vi "Virt.OSC.SUBVI.vi"(0 "VISA resource name":refnum<visa-resource-name>, 11 "Error In":errorcluster) -> (2 "Channel 1 Scale":dbl, 3 "Channel 2 Scale":dbl, 4 "VISA resource name out":refnum<visa-resource-name>, 6 "Time Base":dbl, 8 "vertical trigger":dbl, 10 "horziontal trigger":dbl, 14 "rise/fall":string, 15 "Error Out":errorcluster)   [LabVIEW 2017]
uses:
  <instrlib>/Tektronix TDS 200 1000 2000 Series/Tektronix TDS 200 1000 2000 Series.lvlib
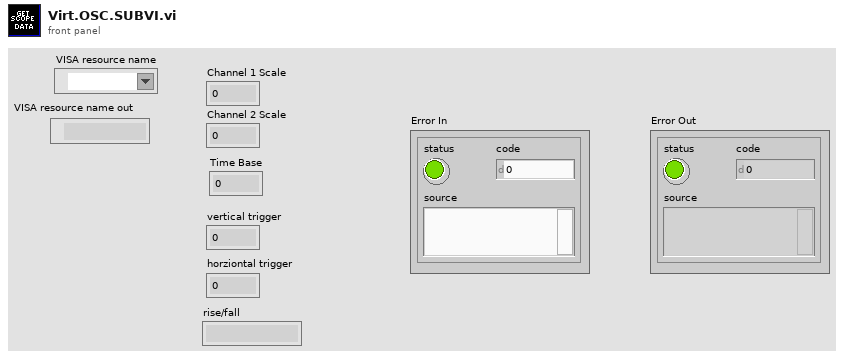
[diagram p1: front panel]
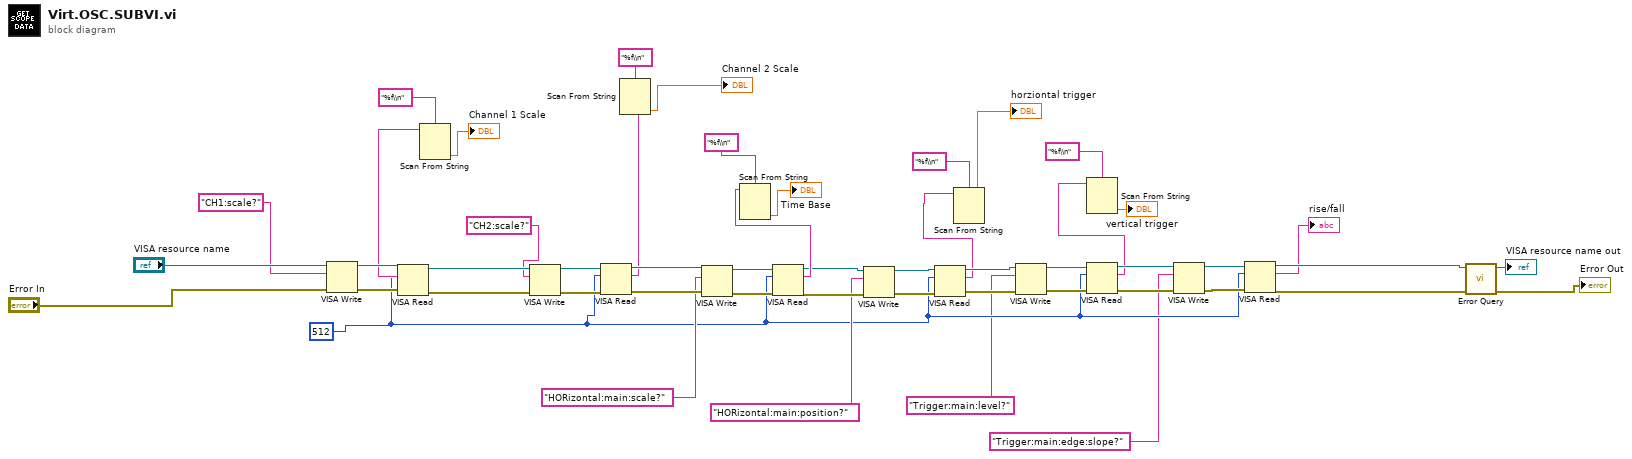
[diagram p0: block diagram]
diagram:
  w10 = 512
  n1 = VISA Write(VISA resource name="VISA resource name", write buffer="CH1:scale?" ("format string"), error in (no error)="Error In") -> (VISA resource name out=w44:refnum<visa-resource-name>, error out=w39:errorcluster)  [unwired: 1 out]
  n2 = VISA Read(VISA resource name=w44, byte count=w10, error in (no error)=w39) -> (VISA resource name out=w43:refnum<visa-resource-name>, read buffer=w34:string, error out=w38:errorcluster)  [unwired: 1 out]
  n3 = Scan From String(format string="%f\\n", input string=w34) -> (output 1=→"Channel 1 Scale":dbl)  [unwired: 2 in, 4 out]
  n4 = VISA Write(VISA resource name=w43, write buffer="CH2:scale?" ("format string"), error in (no error)=w38) -> (VISA resource name out=w42:refnum<visa-resource-name>, error out=w37:errorcluster)  [unwired: 1 out]
  n5 = VISA Read(VISA resource name=w42, byte count=w10, error in (no error)=w37) -> (VISA resource name out=w41:refnum<visa-resource-name>, read buffer=w33:string, error out=w36:errorcluster)  [unwired: 1 out]
  n6 = Scan From String(format string="%f\\n", input string=w33) -> (output 1=→"Channel 2 Scale":dbl)  [unwired: 2 in, 4 out]
  n7 = VISA Write(VISA resource name=w41, write buffer="HORizontal:main:scale?" ("format string"), error in (no error)=w36) -> (VISA resource name out=w40:refnum<visa-resource-name>, error out=w35:errorcluster)  [unwired: 1 out]
  n8 = VISA Read(VISA resource name=w40, byte count=w10, error in (no error)=w35) -> (VISA resource name out=w25:refnum<visa-resource-name>, read buffer=w32:string, error out=w12:errorcluster)  [unwired: 1 out]
  n9 = Scan From String(format string="%f\\n", input string=w32) -> (output 1=→"Time Base":dbl)  [unwired: 2 in, 4 out]
  n10 = VISA Write(VISA resource name=w25, write buffer="HORizontal:main:position?", error in (no error)=w12) -> (VISA resource name out=w24:refnum<visa-resource-name>, error out=w13:errorcluster)  [unwired: 1 out]
  n11 = VISA Read(VISA resource name=w24, byte count=w10, error in (no error)=w13) -> (VISA resource name out=w23:refnum<visa-resource-name>, read buffer=w9:string, error out=w14:errorcluster)  [unwired: 1 out]
  n12 = Scan From String(format string="%f\\n", input string=w9) -> (output 1=→"horziontal trigger":dbl)  [unwired: 2 in, 4 out]
  n13 = VISA Write(VISA resource name=w23, write buffer="Trigger:main:level?", error in (no error)=w14) -> (VISA resource name out=w22:refnum<visa-resource-name>, error out=w15:errorcluster)  [unwired: 1 out]
  n14 = VISA Read(VISA resource name=w22, byte count=w10, error in (no error)=w15) -> (VISA resource name out=w21:refnum<visa-resource-name>, read buffer=w7:string, error out=w16:errorcluster)  [unwired: 1 out]
  n15 = Scan From String(format string="%f\\n", input string=w7) -> (output 1=→"vertical trigger":dbl)  [unwired: 2 in, 4 out]
  n16 = VISA Write(VISA resource name=w21, write buffer="Trigger:main:edge:slope?", error in (no error)=w16) -> (VISA resource name out=w20:refnum<visa-resource-name>, error out=w17:errorcluster)  [unwired: 1 out]
  n17 = VISA Read(VISA resource name=w20, byte count=w10, error in (no error)=w17) -> (VISA resource name out=w19:refnum<visa-resource-name>, read buffer=→"rise/fall":string, error out=w18:errorcluster)  [unwired: 1 out]
  n18 = call <instrlib>:"Error Query.vi"("error in (no error)"=w18, "VISA resource name"=w19) -> ("error out"=→"Error Out":errorcluster, "VISA resource name out"=→"VISA resource name out":refnum<visa-resource-name>)  [unwired: 8 out]
